vi "Read Configuration Data.vi"(8 "error in (no error)":errorcluster) -> (0 "error out":errorcluster, 3 "MHL Configuration":T1)   [LabVIEW 2015]
uses:
  controls/MHL Configuration.ctl
  support/Boiler System Globals.vi
  <vilib>/Utility/config.llb/NI_LVConfig.lvlib
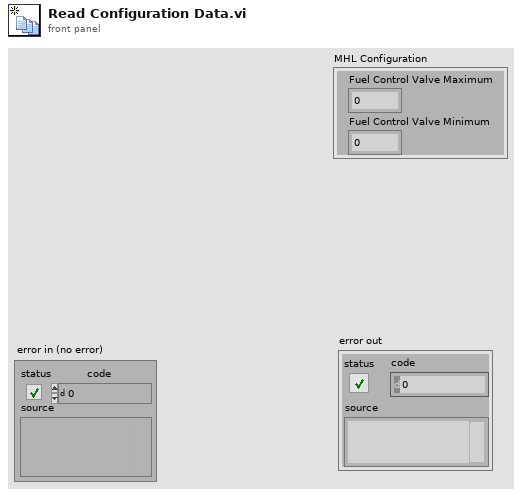
[diagram p1: front panel]
types:
  T1 = typedef "MHL Configuration.ctl" = cluster{"Fuel Control Valve Maximum":dbl, "Fuel Control Valve Minimum":dbl}
  T2 = typedef "NI_LVConfig.lvlib/Config Data RefNum.ctl" = refnum<k1>
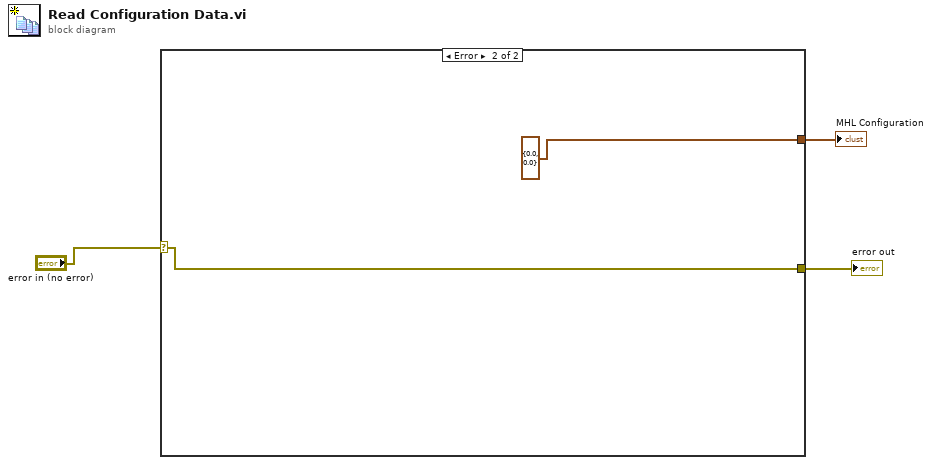
[diagram p0: block diagram]
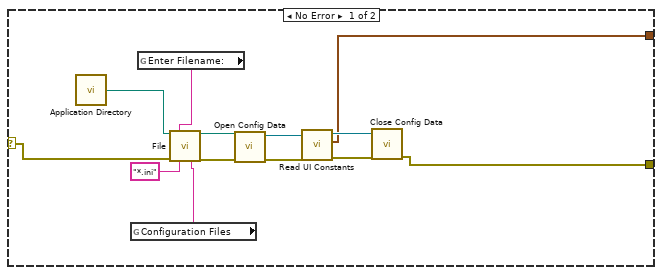
[diagram p2: hidden frame]
diagram:
  n1 = case shown="Error" "error in (no error)" {
    selector: "error in (no error)" -> [w16 w18]
    tunnel: [w10 T1 {"Fuel Control Valve Maximum"=0.0, "Fuel Control Valve Minimum"=0.0} ("MHL Configuration")] -> w2
    tunnel: [w9 w18] -> w1
    frame No Error {
      n2 = call <vilib>:"Application Directory.vi"() -> ("Application Directory"=w7:path)
      n3 = global read "Boiler System Globals.vi" "Configuration Files"() -> (w4:string)
      n4 = global read "Boiler System Globals.vi" "Enter Filename:"() -> (w5:string)
      n5 = call "File"("start path"=w7, "prompt"=w5, "error in"=w16, "pattern (all files)"="*.ini", "pattern label"=w4) -> ("selected path"=w8:path, "error out"=w14:errorcluster)  [unwired: 7 in, 2 out]
      n6 = call <vilib>:"Open Config Data.vi"("error in (no error)"=w14, "configuration file path"=w8) -> ("error out"=w15:errorcluster, "refnum"=w13:T2)  [unwired: 7 in, 1 out]
      n7 = call "Read UI Constants.vi"("error in (no error)"=w15, "CFG File Refun in"=w13) -> ("error out"=w12:errorcluster, "MHL Configuration"=w10:T1, "CFG File Refnum Out"=w11:T2)  [unwired: 7 in]
      n8 = call <vilib>:"Close Config Data.vi"("error in (no error)"=w12, "refnum"=w11) -> ("error out"=w9:errorcluster)  [unwired: 8 in, 1 out]
    }
    frame Error {
    }
  }
  "error out" <- w1
  "MHL Configuration" <- w2
